vi "3JM_Interface.vi"(7 "mode":T1, 8 "error in (no error)":errorcluster caption="에러 입력(에러 없음)", 11 "VISA resource name":refnum<visa-resource-name> caption="Port") -> (0 "error out":errorcluster, 3 "Read":string)   [LabVIEW 2015]
uses:
  3JM_mode.ctl
  <vilib>/Instr/_visa.llb/VISA Configure Serial Port (Serial Instr).vi
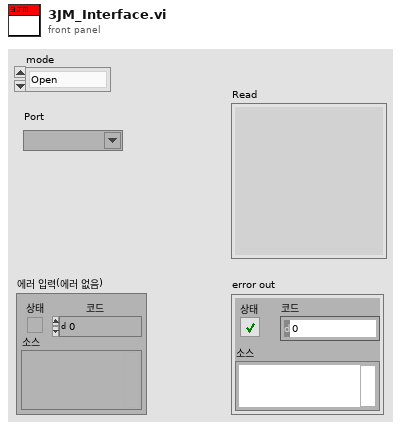
[diagram p1: front panel]
types:
  T1 = typedef "3JM_mode.ctl" = enum16{"Open", "Close", "Read"}
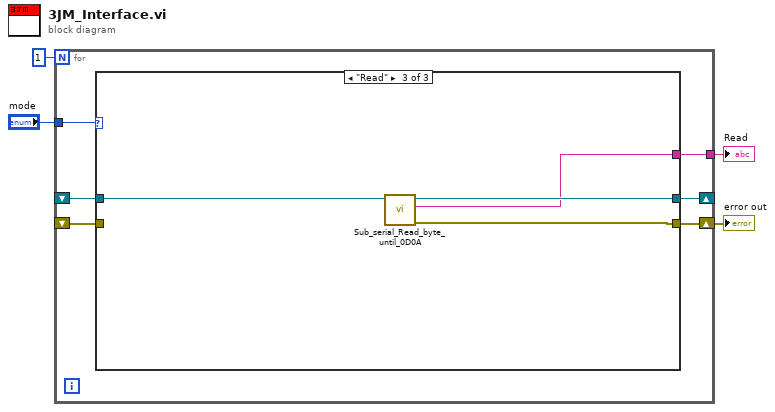
[diagram p0: block diagram]
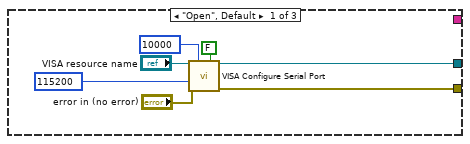
[diagram p2: hidden frame]
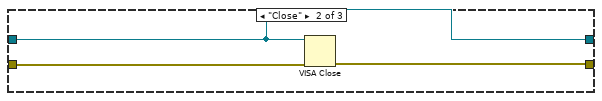
[diagram p3: hidden frame]
diagram:
  n1 = for {
    N: 1 -> [_]
    tunnel: "mode" -> [w10]
    shift-right: [w9] -> _
    shift-left: _ -> [w7]
    shift-right: [w8] -> w2
    shift-left: _ -> [w6]
    tunnel: [w5] -> w1
    n2 = case shown="\"Read\"" w10 {
      tunnel: [w13 w19 w24] -> w9
      tunnel: [w12 w18 w23] -> w8
      tunnel: w7 -> [_ w19 w21]
      tunnel: w6 -> [_ w20 _]
      tunnel: [_ _ w22] -> w5
      frame "Open", Default {
        n3 = call-poly "VISA Configure Serial Port"("VISA resource name"="VISA resource name", "timeout (10sec)"=u32 10000, "Enable Termination\nChar (T)"=FALSE ("Enable Termination\nChar (T)"), "baud rate (9600)"=u32 115200, "error in (no error)"="error in (no error)") -> ("VISA resource name out"=w13:refnum<visa-resource-name>, "error out"=w12:errorcluster)  [unwired: 9 in]
      }
      frame "Close" {
        n4 = VISA Close(VISA resource name=w19, error in (no error)=w20) -> (error out=w18:errorcluster)
      }
      frame "Read" {
        n5 = call "Sub_serial_Read_byte_until_0D0A.vi"("VISA 참조 번호 입력"=w21) -> ("에러 출력"=w23:errorcluster, "버퍼 읽기"=w22:string, "VISA 참조 번호 출력"=w24:refnum<visa-resource-name>)  [unwired: 8 in]
      }
    }
  }
  "error out" <- w2
  "Read" <- w1
